vi "ProcessStartGui.vi"() -> (2 "ok":bool, 3 "repeat?":bool)   [LabVIEW 2016]
uses:
  InfoGui.Action.ctl
  tools/Translator/Translator.Message.ctl
  tools/Translator/Translator.FormatMessage.vi
  Station/Station.Global.vi
  Sequence/Sequence.Global.vi
  tools/Translator/Translator.Global.vi
  Global/ApplicationGlobal.vi
panel:
  out "_loop":i32(ring)=4
  in  "WeekNumber":u16(ring) caption="Numer tygodnia" items=["2118", "2218"]
  in  "CancelButton":bool
  out "Message":string
  out "Status":string
  out "Plate":picture
  in  "ContinueButton":bool
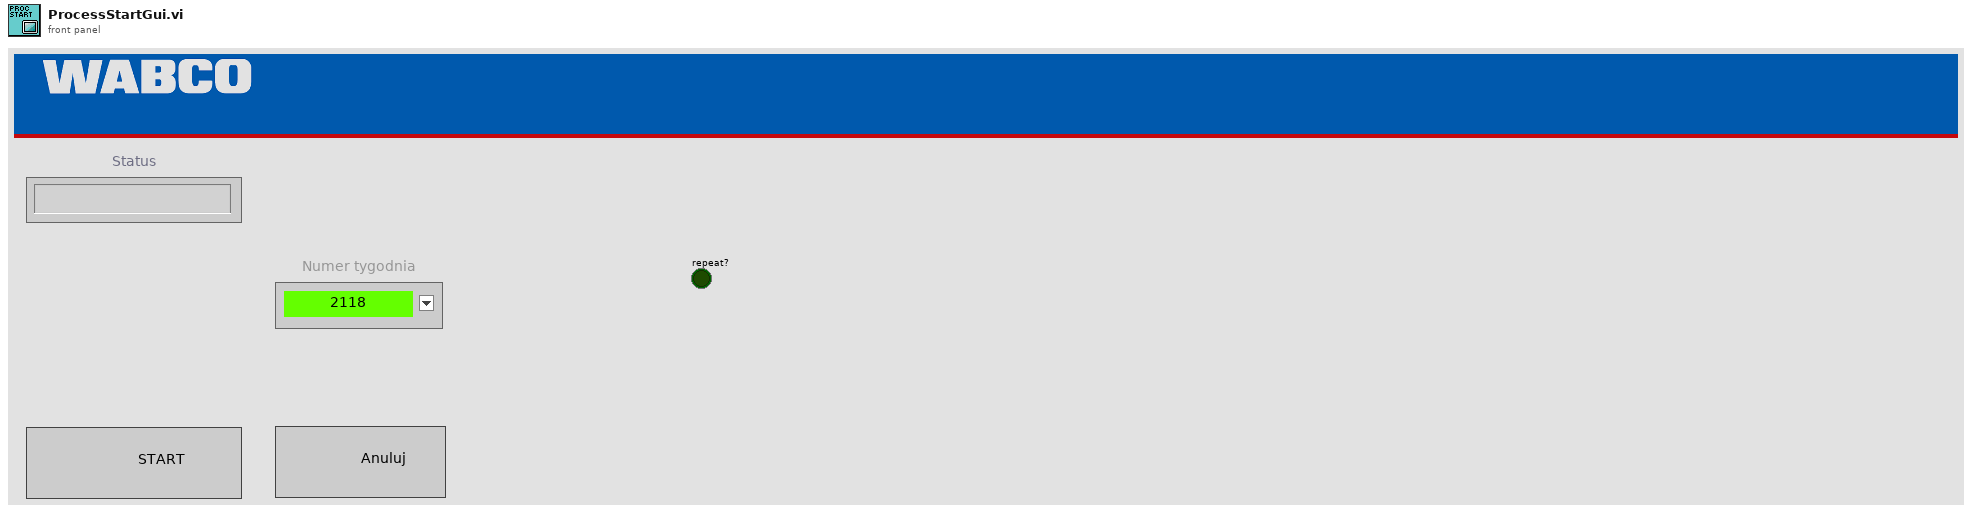
[diagram p1: front panel]
types:
  T1 = typedef "InfoGui.Action.ctl" = enum32{"idle", "constructor", "destructor", "--- InfoGUI ---"}
  T2 = typedef "Translator.Message.ctl" = enum16{"-", "Event confirmed", "Log out", "Log in", "Shutdown", "Cancel", "Start", "Begin time", "End time", "Duration", "Service Mode", "Ignore Results", "Serial Format", "On", "Off", "OK", "NOK", "NOK %s", "Home", "Work", "Close", "Open", "In progress...", "Missing", "Empty", "Hardware failure", "Initial", "Default", "Total", "Out of range", "Free disk space is below 1GB - contact technician", "Error %d >> %s", "Error %d >> %s >> %s", "Msg %d >> %s", "Laser msg %d %s", "Laser cmd error %s %d", "Laser cmd failed %s", "Laser cmd warning %s", "Laser disconnected", "Laser status %s", "Laser already started", "Laser job unkonwn %s", "Laser job missing %s", "Laser job select failure %s", "Unable to start laser printing (%s)", "Unable to stop laser printing (%s)", "Laser marking aborted", "Laser marking timeout", "Unable to reset Laser Interlock (%s)", "Unable to trigger Laser. Laser not ready (%s)", "Laser job '%s' coordinates not configured", "Starting %s", "Quitting %s", "Configured", "Initializing", "Quitting", "Loading", "Loaded %d results", "Loaded %d events", "Running", "Stopped", "Summary", "Laser", "Do you want to continue?", "Do you want to delete the configuration?", "The configuration is being used by an order. Unable to delete!", "Press confirm button", "Station is not based. Do you want to exit?", "Station requires changeover. Do you want to run the test?", "Test options are not set as default. Do you want to continue?", "Formatting of WabcoNo is disabled. Do you want to continue?", "Product not detected. Do you want to continue?", "Product scan failed. Do you want to continue?", "Calibration", "Log out?", "System", "All", "IDLE", "Translating...%s", "Not found", "Alarm %s", "Run", "Skip", "Abort", "Repeat", "Please wait...", "Database disconnected", "Database disconnected - changeover disabled!", "Login to database successful", "Login to database failed: %d; %s", "Unable to check the product status of reference %d - database disconnected", "Unable to set the product status of reference %d - database disconnected", "Variant file backup %s", "Read variant (%s)", "Result", "Station armed!", "Station requires changeover!", "Select reference number...", "EMERGENCY BUTTON - press Control button", "EMERGENCY DOOR - press Control button", "Resetting Emergency...", "Unable to reset safety circuit - Emergency Button pressed", "Unable to reset safety circuit - Emergency Side Door open", "Station not based", "Station based", "Station not empty", "Station basing...", "No order", "Press Start to begin new order", "Scanning new order", "Order NOK. Correct or scan again", "Order OK. Press Accept", "Order ready", "Revolver incorrect", "Fork incorrect", "Revolver missing", "Revolver empty", "Container missing", "Offline results", "Offline statistics", "Updating statistics %.1f %%", "DMC Configurator", "Door open", "Close the front door", "Press start button", "Done. Open the front door", "Running...", "Running...%.1f %%", "Pause %s", "Pause %s. NOK container missing", "Pause %s. OK container missing", "Pause %s. Revolver empty", "Pause %s. Revolver missing", "Pause %s. Revolver incorrect", "Pause %s. Fork missing", "Pause %s. Fork incorrect", "Pause %s. Too many failures", "Pause %s. Unloading failure", "Pause %s. One slot is not working", "Pause %s. Part order is done. Empty OK container", "Pause %s. Unable to move product to slot", "Pause %s. Unable to move back product pusher", "Pause %s. Unable to lift product", "Pause %s. Unable to move back product lifter", "Pause %s. Unable to move product arm to Work", "Pause %s. Unable to move product arm to NOK", "Pause %s. Unable to move product arm to OK", "Pause %s. Unable to unsuck the NOK product", "Pause %s. Unable to drop the NOK product", "Pause %s. Product OK missing", "Pause %s. Unable to unsuck the OK product", "Pause %s. Unable to drop the OK product", "Stopping...", "File '%s' is missing", "File '%s' is broken", "File '%s' is running", "Log file started (%s)", "Log file ended (%s)", "Log file stopped (%s)", "Log file ignored (%s)", "Log file exported (%s)", "Log file export failed (%s)", "Wrong serial number in log file", "Wrong reference number in log file", "Test steps are missing", "%s = %.3f", "Process param '%s' not found in DB", "Process param '%s' wrong order", "Process param '%s' value %.3f out of limits (%.3f; %.3f)", "Step%d param '%s' not found in DB", "Step%d param '%s' wrong order", "Step%d param '%s' value %.3f out of limits (%.3f; %.3f)", "Step%d EV '%s' not found in DB", "Step%d EV '%s' wrong order", "\"%s\" not found in DB", "\"%s\" wrong order", "\"%s\" value %.3f out of limits (%.3f; %.3f)", "\"%s\" not found in software", "Process init (%s)", "Process started", "Process restarted", "Process run", "Process done", "Process done - remove OK container", "Process aborted", "Process aborted at work", "Process aborted at home", "Process error", "Process error at home", "Process error at work", "Process close", "Process pause", "Process continue", "Process door open", "Process door close", "Process pause at slot %s due to %s", "Select plate from the order to process", "Do you want to start the process?", "Do you want to continue the process?", "There is unfinished order. Do you want to put the new order?", "Product %s %d OK", "Product %s %d NOK", "Unable to unload the slot %s. Product missing in the slot", "Unable to unload the slot %s. Product already in the arm", "Unable to accept the product as OK. Product missing in slot %s", "Unable to accept the product as OK. Product could not drop into the container at slot %s", "Unable to accept the product as NOK. Product could not drop into the container at slot %s", "Scan failed. Error %s", "Scan failed. Scanner disconnected", "Scan failed. Wrong Wabco number %d, limit (%d,%d)", "Scan failed. Wrong serial number %d, limit (%d,%d)", "Scan failed. Wrong date %d, limit (%d,%d)", "Scan failed. Wrong product wabco number %d (expected %d)", "Scan failed. Wrong product serial number %d (expected > 0)", "Scan OK %s", "Scan failed. Unable to determine table position (%s)", "Scan failed. Timeout", "Tune failed. Scanner disconnected", "Tune failed. Timeout", "%s = %d", "%s = %d->%d", "Unable to set %s = %.2f - Air Pressure Inside off", "Unable to set digital output '%s' = %d", "Unable to activate air pressure inside - timeout", "Unable to activate air pressure inside - aborted", "Unable to switch on Air Main Valve - Air Pressure Inlet off", "Unable to switch on Air Main Valve - Door open", "Unable to switch off Air Main Valve - timeout", "Unable to switch off Air Main Valve - aborted", "Unable to rotate Table - timeout", "Unable to rotate Table - aborted", "Unable to rotate Table - Product Move not in Home position", "Unable to rotate Table - Air Pressure Inside off", "Unable to rotate Table - Product Lift A not in Home position", "Unable to rotate Table - Product Lift B not in Home position", "Unable to rotate Table - unlock before movement timeout", "Unable to rotate Table - lock after movement timeout", "Unable to move Table Lock to %s position - timeout", "Unable to move Table Lock to %s position - aborted", "Unable to move Table Lock to %s position - Air Pressure Inside off", "Unable to move Table Lock to %s position - Table not in position", "Unable to move Product Lift A to %s position - timeout", "Unable to move Product Lift B to %s position - timeout", "Unable to move Product Lift A to %s position - aborted", "Unable to move Product Lift B to %s position - aborted", "Unable to move Product Lift A to %s position - Air Pressure Inside off", "Unable to move Product Lift B to %s position - Air Pressure Inside off", "Unable to move Product Lift A to %s position - Table not locked", "Unable to move Product Lift B to %s position - Table not locked", "Unable to move Product Lift A to %s position - Product Arm not in Work position", "Unable to move Product Lift B to %s position - Product Arm not in Work position", "Unable to set Product Suction Gripper %s to %s - timeout", "Unable to set Product Suction Gripper %s to %s - aborted", "Unable to set Product Suction Gripper %s to %s - Air Pressure Inside off", "Unable to set Product Suction Gripper %s to %s - Table slot unkown", "Unable to move Product Arm to %s position - timeout", "Unable to move Product Arm to %s position - aborted", "Unable to move Product Arm to %s position - Air Pressure Inside off", "Unable to move Product Arm to %s position - Product Lift A not in Home position", "Unable to move Product Arm to %s position - Product Lift B not in Home position", "Unable to move Product to %s position - timeout", "Unable to move Product to %s position - aborted", "Unable to move Product to %s position - Air Pressure Inside off", "Unable to move Product to %s position - Table not in position"}
  T3 = typedef "FestoCPX.Station.ButtonsState.ctl" = cluster{"Start":bool, "Stop":bool, "Control":bool}
  T4 = typedef "Sequence.Data.ctl" = cluster{"BeginTS":timestamp, "EndTS":timestamp, "State":T5, "Status.Work":T6, "Status.Process":T6, "Status.Home":T6, "Status.Wabco":T6, "Status.Client":T6, "BreakReason":T7, "BreakSource":T8, "DoorLock":bool, "Status.Prod":T9[], "UserAction":T13, "UserData":T14, "Error":errorcluster, "Code":T17, "Rotations":i32, "ProdIdx":i32, "ProdDone":T9[], "PrintedSerials-Wabco":i32[], "PrintedSerials-Client":i32[], "Counters-Wabco":T24, "Counters-Client":T24}
  T5 = typedef "Sequence.State.ctl" = enum16{"Init", "Idle", "Home", "Work", "Run", "Pause"}
  T6 = typedef "Sequence.Step.Status.ctl" = enum16{"-", "Pending", "Running", "Skipped", "Passed", "Failed", "Done", "Error", "Aborted", "Stopped"}
  T7 = typedef "Sequence.Test.BreakReason.ctl" = enum16{"-", "NOK container", "OK container", "Rev empty", "Rev missing", "Rev wrong", "Fork missing", "Fork wrong", "NOK limit", "Unload failure", "Single slot", "Part done", "Err: Prod move work", "Err: Prod move home", "Err: Prod lift work", "Err: Prod lift home", "Err: Prod Arm Work", "Err: Prod Arm NOK", "Err: Prod Arm OK", "Err: Prod NOK suck", "Err: Prod NOK drop", "Err: Prod OK missing", "Err: Prod OK suck", "Err: Prod OK drop"}
  T8 = typedef "Sequence.Test.BreakSource.ctl" = enum16{"-", "A", "B", "A/B"}
  T9 = typedef "Sequence.Test.Status.ctl" = cluster{"Slot":T10, "A":T12, "B":T12}
  T10 = typedef "Sequence.Slot.StatusData.ctl" = cluster{"ID":i32, "Unload":T11, "TS":timestamp, "duration":u32}
  T11 = typedef "Sequence.Test.Unload.Status.ctl" = enum16{"init", "check NOK", "check OK", "wait on NOK", "wait on OK", "wait on Unload", "done"}
  T12 = typedef "Sequence.Prod.StatusData.ctl" = cluster{"status":T6, "pause":T7, "present":bool, "printed":bool, "scanned":bool, "tuned":bool, "removed":bool, "serial":i32, "code":string, "path":path, "corners":cluster{"X":i32, "Y":i32}[], "verification":u8}
  T13 = typedef "Sequence.UserActions.ctl" = cluster{"Stop":bool, "Pause":bool, "Next":bool}
  T14 = typedef "Sequence.UserData.ctl" = cluster{"GuiMode":T15, "Test":T16, "ContinueOrder":bool}
  T15 = typedef "Sequence.MainMode.ctl" = enum16{"Process", "Base", "Order", "Manual", "Logs", "Results", "Stats", "DMC Config"}
  T16 = typedef "MainGui.TestOptions.ctl" = cluster{"IgnoreResults":bool, "IgnoreImages":bool, "ServiceMode":bool}
  T17 = typedef "Sequence.Code.Sets.ctl" = cluster{"Ready":bool, "DoubleOrder":bool, "OrderDone":bool, "AllowSingleSlot":bool, "TunedA":bool, "TunedB":bool, "CheckDM":bool, "ThresholdA":u8, "ThresholdB":u8, "Plate":T18, "ImgPath":path, "Variant":T19}
  T18 = typedef "Sequence.PlateType.ctl" = enum16{"Wabco", "Client"}
  T19 = typedef "Logger.Variant.Sets.ctl" = cluster{"State":T20, "ImgPath":path, "WabcoPlate":string, "WabcoProduct":string, "ClientProduct":string, "ClientPlate":string, "TotalQuantity":u16, "OrderQuantity":u16, "Serial":i32, "Wabco":T21, "Client":T21}
  T20 = typedef "Station.Changeover.State.vi" = enum16{"Init", "Scaning", "NOK", "Wait for ack", "Ready"}
  T21 = typedef "Station.Plate.Properties.ctl" = cluster{"LaserJob":string, "AdditionalTxt":string, "FactoryCode":string, "RevID":u8, "ForkID":u8, "FailuresLimit":u16, "GlobalCnt":i32, "Bank":u8, "SerialFormat":T22, "CoordA":T23, "CoordB":T23, "DMCconfig":i32}
  T22 = typedef "Sequence.Code.SerialFormat.ctl" = enum8{"", "6 dig", "7 dig"}
  T23 = typedef "V7310.Job.Sets.ctl" = cluster{"X":dbl, "Y":dbl, "Angle":dbl}
  T24 = typedef "Sequence.Counters.ctl" = cluster{"Expected":u16, "Done":u16, "OK":u16, "NOK":u16, "NOKlimit":u16, "Part":u16, "PartOK":u16}
  T25 = typedef "LVPositionTypeDef.ctl" = cluster{"Left":i32, "Top":i32}
  T26 = typedef "imagedata.ctl" = cluster{"image type":i32, "image depth":i32, "image":u8[], "mask":u8[], "colors":u32[], "Rectangle":cluster{"left":i16, "top":i16, "right":i16, "bottom":i16}}
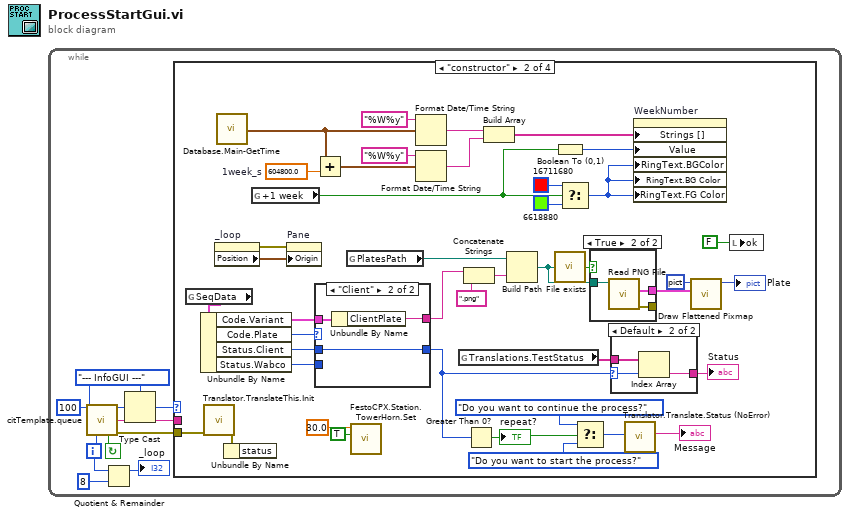
[diagram p0: block diagram]
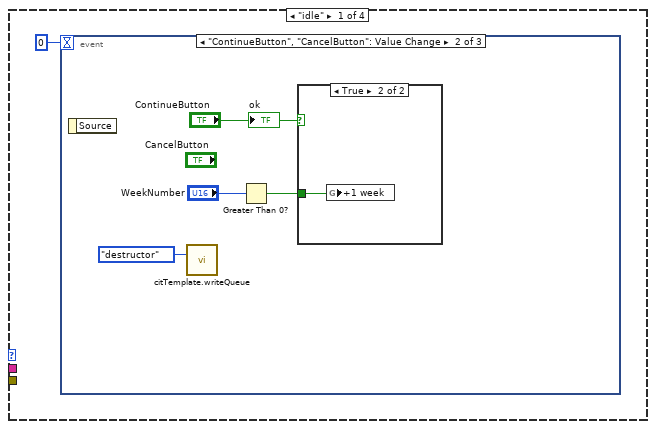
[diagram p2: hidden frame]
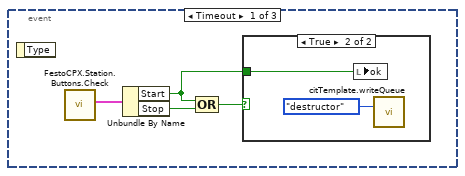
[diagram p3: hidden frame]
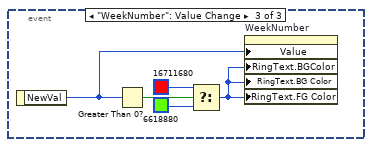
[diagram p6: hidden frame]
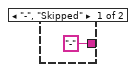
[diagram p7: hidden frame]
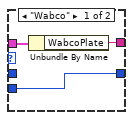
[diagram p8: hidden frame]
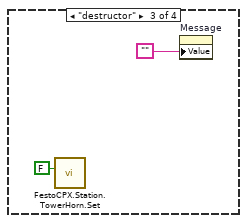
[diagram p10: hidden frame]
diagram:
  n1 = while {
    i -> [w1]
    stop <- w10 continue-if-true
    w4 = InfoGui.Action."--- InfoGUI ---" ("Action")
    n2 = call "citTemplate.queue.vi"("ms timeout (250 ms)"=100, "event enum"=w4, "iteration (-1)"=w1) -> ("event out"=w8:u32, "(flatten) data out"=w5:string, "continue"=w10:bool, "error out"=w6:errorcluster)  [unwired: 2 in, 7 out]
    n3 = Quotient & Remainder(x=w1, y=8) -> (x-y*floor(x/y)=→"_loop":i32)  [unwired: 1 out]
    n4 = Type Cast(type=w4, x=w8) -> (*(type *) &x=w7:T1)
    n5 = case shown="\"constructor\"" w7 {
      tunnel: w6 -> [_ w42 _ _]
      tunnel: w5 -> [_ _ _ _]
      frame "idle" {
        n6 = event shown="[1] \"ContinueButton\", \"CancelButton\": Value Change" {
          selector: _ -> [_ _ _]
          dyn-events: _ -> [_ _ _]
          timeout: 0 -> [_ _ _]
          event Timeout {
            n7 = event-data() -> ()  [unwired: 2 out]
            n8 = call "FestoCPX.Station.Buttons.Check.vi"() -> ("Buttons.State"=w15:T3)  [unwired: 10 in, 1 out]
            n9 = Unbundle By Name(w15) -> ("Start"=w12:bool, "Stop"=w14:bool)
            n10 = Compound Arithmetic op=OR(w12, w14) -> (w13:bool)
            n11 = case shown="True" w13 {
              tunnel: w12 -> [_ w16]
              frame False {
              }
              frame True {
                n12 = local write "ok"(w16) -> ()
                n13 = call "citTemplate.writeQueue.vi"("event in (if not connected:all statemachine with data event)"=InfoGui.Action."destructor" ("Action")) -> ()  [unwired: 14 in, 1 out]
              }
            }
          }
          event "ContinueButton", "CancelButton": Value Change {
            n14 = event-data() -> ()  [unwired: 2 out]
            n15 = call "citTemplate.writeQueue.vi"("event in (if not connected:all statemachine with data event)"=InfoGui.Action."destructor" ("Action")) -> ()  [unwired: 14 in, 1 out]
            n16 = Greater Than 0?(x="WeekNumber") -> (x > 0?=w19:bool)
            n17 = case shown="True" "ContinueButton" {
              tunnel: w19 -> [_ w22]
              frame False {
              }
              frame True {
                n18 = global write "Station.Global.vi" "+1 week"(w22) -> ()
              }
            }
            "ok" <- "ContinueButton"
          }
          event "WeekNumber": Value Change {
            n19 = event-data() -> ("NewVal"=w23:u16)  [unwired: 1 out]
            n20 = Greater Than 0?(x=w23) -> (x > 0?=w24:bool)
            n21 = Select(t=u32 16711680, s=w24, f=u32 6618880) -> (s? t:f=w27:u32)
            n22 = property on="WeekNumber" class="Ring (strict)"("Value"=w23, "RingText.BGColor"=w27, "RingText.BG Color"=w27, "RingText.FG Color"=w27) -> ()  [unwired: 2 in, 2 out]
          }
        }
      }
      frame "constructor" {
        w30 = 604800.0  # 1week_s
        n23 = global read "Sequence.Global.vi" "SeqData"() -> (w52:T4)
        n24 = Unbundle By Name(w52) -> ("Code.Variant"=w68:T19, "Code.Plate"=w51:T18, "Status.Client"=w50:T6, "Status.Wabco"=w49:T6)
        n25 = call "Translator.TranslateThis.Init.vi"("error in"=w42) -> ("error out"=w41:errorcluster)  [unwired: 10 in]
        n26 = property on="_loop" class="Ring (strict)"() -> (error out=w59:errorcluster, "Position"=w60:T25)  [unwired: 2 in, 1 out]
        n27 = call "Database.Main-GetTime.vi"() -> ("TS"=w28:timestamp)  [unwired: 1 in]
        n28 = Unbundle By Name(w41) -> ()  [unwired: 1 out]
        n29 = global read "Station.Global.vi" "+1 week"() -> (w39:bool)
        n30 = property on="Pane" class="Pane"(error in=w59, "Origin"=w60) -> ()  [unwired: 1 in, 2 out]
        n31 = Add(x=w28, y=w30) -> (x+y=w31:timestamp)
        n32 = case shown="\"Client\"" w51 {
          tunnel: w68 -> [w75 w79]
          tunnel: [w74 w78] -> w48
          tunnel: w50 -> [_ w77]
          tunnel: [w76 w77] -> w46
          tunnel: w49 -> [w76 _]
          frame "Wabco" {
            n33 = Unbundle By Name(w75) -> ("WabcoPlate"=w74:string)
          }
          frame "Client" {
            n34 = Unbundle By Name(w79) -> ("ClientPlate"=w78:string)
          }
        }
        n35 = global read "ApplicationGlobal.vi" "PlatesPath"() -> (w69:path)
        n36 = call "FestoCPX.Station.TowerHorn.Set.vi"("Horn (F)"=TRUE ("Horn1 (F)"), "Period [s] (0)"=30.0) -> ()  [unwired: 9 in, 1 out]
        n37 = Format Date/Time String(time format string (%c)="%W%y", seconds (now)=w28) -> (date/time string=w33:string)  [unwired: 1 in]
        n38 = Format Date/Time String(time format string (%c)="%W%y", seconds (now)=w31) -> (date/time string=w34:string)  [unwired: 1 in]
        n39 = global read "Translator.Global.vi" "Translations.TestStatus"() -> (w47:string[])
        n40 = Concatenate Strings(w48, ".png" ("string")) -> (w65:string)
        n41 = Greater Than 0?(x=w46) -> (x > 0?=w57:bool)
        "repeat?" <- w57
        n42 = Build Array(w33, w34) -> (w35:string[])
        n43 = Build Path(base path=w69, name or relative path=w65) -> (appended path=w64:path)
        n44 = Boolean To (0,1)(Boolean=w39) -> (0, 1=w36:i16)
        n45 = call "File exists.vi"("file path"=w64) -> ("exists?"=w63:bool)  [unwired: 4 in]
        n46 = Select(t=u32 16711680, s=w39, f=u32 6618880) -> (s? t:f=w40:u32)
        n47 = Select(t=Translator.Message."Do you want to continue the process?" ("_Msg"), s=w57, f=Translator.Message."Do you want to start the process?" ("_Msg")) -> (s? t:f=w54:T2)
        n48 = case shown="True" w63 {
          tunnel: w64 -> [_ w82]
          tunnel: [_ w81] -> w61
          tunnel: [_ w80] -> _
          frame False {
          }
          frame True {
            n49 = call <vilib>:"Read PNG File.vi"("path to PNG file"=w82) -> ("error out"=w80:errorcluster, "image data"=w81:T26)  [unwired: 8 in, 1 out]
          }
        }
        n50 = case shown="Default" w46 {
          selector: w46 -> [_ w72]
          tunnel: ["-" ("String") w71] -> w45
          tunnel: w47 -> [_ w73]
          frame "-", "Skipped" {
          }
          frame Default {
            n51 = Index Array(array=w73, index=w72) -> (element=w71:string)
          }
        }
        "Status" <- w45
        n52 = call "Translator.Translate.Status (NoError).vi"("msg"=w54) -> ("Translated Msg"=→"Message":string)  [unwired: 10 in]
        n53 = property on="WeekNumber" class="Ring (strict)"("Strings []"=w35, "Value"=w36, "RingText.BGColor"=w40, "RingText.BG Color"=w40, "RingText.FG Color"=w40) -> ()  [unwired: 2 in, 2 out]
        n54 = call <vilib>:"Draw Flattened Pixmap.vi"("image data"=w61, "picture"=picture data[5B]) -> ("new picture"=→"Plate":picture)  [unwired: 7 in]
        n55 = local write "ok"(FALSE ("_b_ok")) -> ()
      }
      frame "destructor" {
        n56 = call "FestoCPX.Station.TowerHorn.Set.vi"("Horn (F)"=FALSE ("Horn1 (F)")) -> ()  [unwired: 10 in, 1 out]
        n57 = property on="Message" class="Str"("Value"="") -> ()  [unwired: 2 in, 2 out]
      }
      frame "--- InfoGUI ---" {
      }
    }
  }
